vi "Experiment_3D_drawing.vi"() -> ()   [LabVIEW 2023]
uses:
  <vilib>/picture/3D Picture Control/Object/Create Object (drawable).vi
  <vilib>/picture/3D Picture Control/NI_3D Picture Control.lvlib
panel:
  in  "Axis":cluster{"X":sgl, "Y":sgl, "Z":sgl}
  in  "Angle":sgl
  out "3D Picture":refnum<vi>(3d-picture)
  in  "error in (no error)":errorcluster
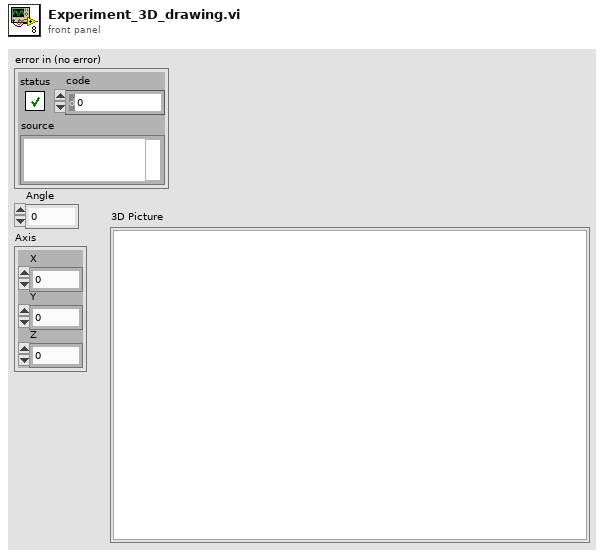
[diagram p1: front panel]
types:
  T1 = cluster{"Red":sgl, "Green":sgl, "Blue":sgl, "Alpha":sgl}
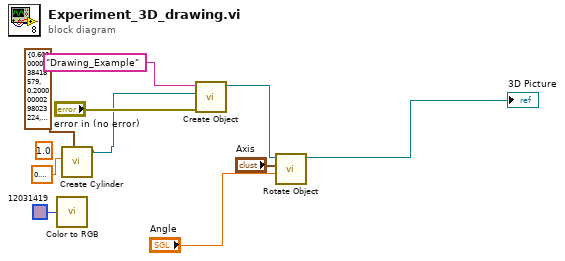
[diagram p0: block diagram]
diagram:
  (unwired) sgl 1.0 ("Height")
  n1 = call <vilib>:"Color to RGB.vi"("Color"=u32 12031419) -> ()  [unwired: 4 out]
  n2 = call <vilib>:"Create Cylinder.vi"("Color"=T1 {"Red"=0.6, "Green"=0.2, "Blue"=0.1, "Alpha"=0.5}, "Radius"=sgl 0.2) -> ("New Cylinder Refnum"=w8:refnum<vi>)  [unwired: 8 in, 1 out]
  n3 = call-poly <vilib>:"Create Object.vi"("error in (no error)"="error in (no error)", "Geometry"=w8, "Name"="Drawing_Example") -> ("Scene:New Object"=w6:refnum<vi>)  [unwired: 7 in, 1 out]
  n4 = call <vilib>:"Rotate Object.vi"("Angle"="Angle", "Axis"="Axis", "Scene.Object In"=w6) -> ("Scene.Object Out"=→"3D Picture":refnum<vi>)  [unwired: 7 in, 1 out]
